vi "set_TRIG.vi"   [LabVIEW 2011]
doc: "reads the global variables and configurates TRIG1 & TRIG2 accordingly"
uses:
  global.vi
panel:
  # "see block diagram"
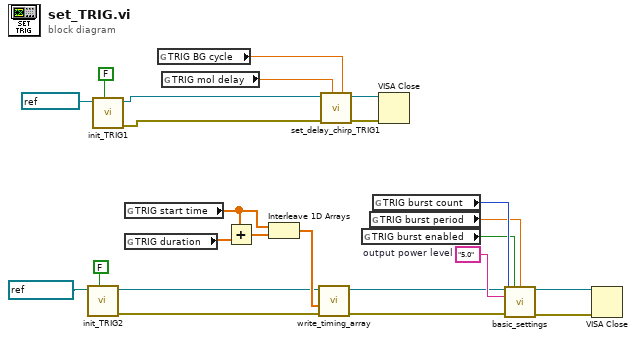
[diagram p0: block diagram]
diagram:
  w21 = "5.0"  # output power level
  n1 = call "init_TRIG2.vi"("reset TRIG"=FALSE, "VISA resource name"=refnum<visa-resource-name> "TRIG2" ("TRIG2 resource name")) -> ("error out"=w7:errorcluster, "VISA resource name out"=w8:refnum<visa-resource-name>)  [unwired: 5 in]
  n2 = call "init_TRIG1.vi"("reset"=FALSE, "VISA resource name"=refnum<visa-resource-name> "TRIG1") -> ("error out"=w12:errorcluster, "VISA resource name out"=w13:refnum<visa-resource-name>)  [unwired: 8 in]
  n3 = global read "global.vi" "TRIG start time"() -> (w10:dbl[])
  n4 = global read "global.vi" "TRIG duration"() -> (w11:dbl[])
  n5 = global read "global.vi" "TRIG BG cycle"() -> (w14:dbl)
  n6 = global read "global.vi" "TRIG mol delay"() -> (w15:dbl)
  n7 = Add(x=w10, y=w11) -> (x+y=w9:dbl[])
  n8 = Interleave 1D Arrays(w10, w9) -> (w20:dbl[])
  n9 = call "write_timing_array.vi"("error in"=w7, "delay array"=w20, "VISA resource in"=w8) -> ("error out 2"=w3:errorcluster, "VISA resource out"=w4:refnum<visa-resource-name>)  [unwired: 3 in]
  n10 = call "set_delay_chirp_TRIG1.vi"("background period"=w14, "molecular delay"=w15, "error in"=w12, "VISA resource name"=w13) -> ("error out"=w5:errorcluster, "VISA resource name out"=w6:refnum<visa-resource-name>)  [unwired: 6 in]
  n11 = global read "global.vi" "TRIG burst enabled"() -> (w23:bool)
  n12 = global read "global.vi" "TRIG burst period"() -> (w22:dbl)
  n13 = global read "global.vi" "TRIG burst count"() -> (w24:i32)
  n14 = VISA Close(VISA resource name=w6, error in (no error)=w5) -> ()  [unwired: 1 out]
  n15 = call "basic_settings.vi"("VISA resource name"=w4, "Burst enable?"=w23, "burst period (s)"=w22, "burst count"=w24, "power level"=w21, "error in (no error)"=w3) -> ("VISA resource name out"=w2:refnum<visa-resource-name>, "error out"=w1:errorcluster)  [unwired: 8 in]
  n16 = VISA Close(VISA resource name=w2, error in (no error)=w1) -> ()  [unwired: 1 out]
